vi "PDF Konfig CG.vi"(8 "error in (no error)":errorcluster caption="Fehler (Eingang, kein Fehler)", 11 "seconds since 1Jan1904":timestamp) -> (0 "error out":errorcluster caption="Fehler (Ausgang)")   [LabVIEW 2020, in "Erweiterte Konfig.lvlib" / "CG-Check Konfig.lvlib"]
uses:
  CG-Check Konfig.lvlib
  Schedule Modul/Aktion FGV Testdaten sammeln.ctl
  Sprachverwaltung/FGV Aktion Tabelle zerlegen.ctl
  Linearisierung V2/Protokoll/Protokoll.lvlib
  Schedule Modul/Schedule Modul.lvlib
  Sprachverwaltung/Sprachverwaltung.lvlib
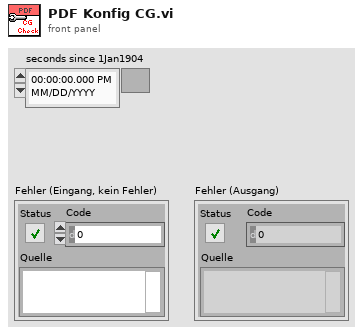
[diagram p1: front panel]
types:
  T1 = typedef "Sprachverwaltung.lvlib/FGV Aktion Tabelle zerlegen.ctl" = enum16{"laden", "vereinzeln", "speichern"}
  T2 = typedef "Schedule Modul.lvlib/Aktion FGV Testdaten sammeln.ctl" = enum16{"lesen", "Dichtheitstest", "CalGasTest", "T90", "Kalibrieren", "init", "Kalender Daten"}
  T3 = typedef "Schedule Modul.lvlib/Ergebnis CalGas Test.ctl" = cluster{"Istwerte":string[][], "Auswertung":string[][][], "Fehler":bool[], "Abweichung in %":string[][], "Spanauswahl":i32[]}
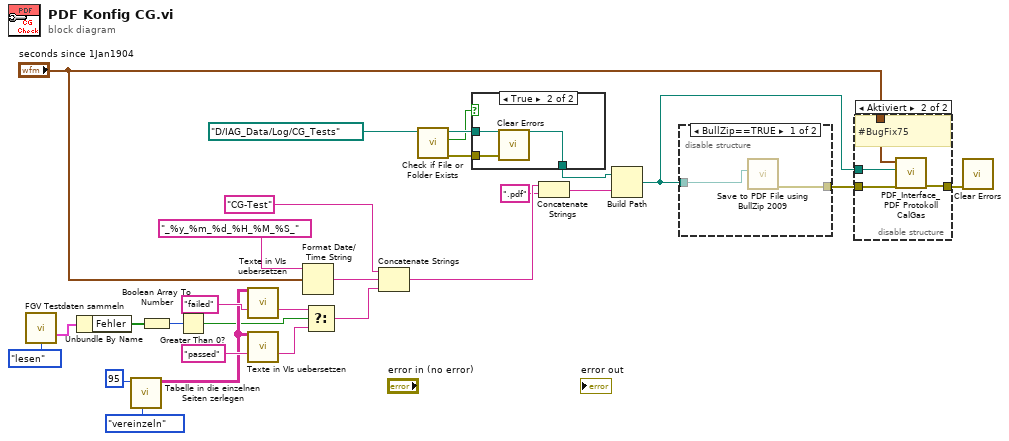
[diagram p0: block diagram]
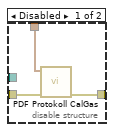
[diagram p2: hidden frame]
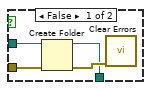
[diagram p3: hidden frame]
diagram:
  n1 = call "FGV Testdaten sammeln.vi"("Aktion"=Aktion_FGV_Testdaten_sammeln."lesen") -> ("Ergebnis CalGas Test"=w16:T3)  [unwired: 9 in, 5 out]
  n2 = Unbundle By Name(w16) -> ("Fehler"=w15:bool[])
  n3 = call "Tabelle in die einzelnen Seiten zerlegen.vi"("Aktion"=FGV_Aktion_Tabelle_zerlegen."vereinzeln", "Index (Seite)"=95) -> ("Sprachliste"=w4:string[][])  [unwired: 7 in, 2 out]
  n4 = Boolean Array To Number(Boolean array=w15) -> (number=w14:u32)
  n5 = Greater Than 0?(x=w14) -> (x > 0?=w3:bool)
  n6 = call "Texte in VIs uebersetzen.vi"("Sprachliste"=w4, "String zum Übersetzen"="failed" ("String")) -> ("String zum Übersetzen"=w6:string)  [unwired: 9 in, 4 out]
  n7 = call "Texte in VIs uebersetzen.vi"("Sprachliste"=w4, "String zum Übersetzen"="passed" ("String")) -> ("String zum Übersetzen"=w5:string)  [unwired: 9 in, 4 out]
  n8 = Format Date/Time String(time format string (%c)="_%y_%m_%d_%H_%M_%S_" ("Zeitformatierungs-String (%c)"), seconds (now)="seconds since 1Jan1904") -> (date/time string=w21:string)  [unwired: 1 in]
  n9 = Select(t=w6, s=w3, f=w5) -> (s? t:f=w2:string)
  n10 = Concatenate Strings("CG-Test" ("String"), w21, w2) -> (w23:string)
  n11 = call <vilib>:"Check if File or Folder Exists.vi"("path"=path "D:/IAG_Data/Log/CG_Tests" ("Pfad:")) -> ("error out"=w28:errorcluster, "file or folder exists?"=w25:bool, "dup path"=w26:path)  [unwired: 8 in]
  n12 = case shown="True" w25 {
    tunnel: w26 -> [w32 w34]
    tunnel: [w30 w34] -> w27
    tunnel: w28 -> [w29 w33]
    frame False {
      n13 = Create Folder(path (use dialog)=w32, error in=w29) -> (created path=w30:path, error out=w31:errorcluster)  [unwired: 1 in, 1 out]
      n14 = call <vilib>:"Clear Errors.vi"("error in (no error)"=w31) -> ()  [unwired: 5 in, 2 out]
    }
    frame True {
      n15 = call <vilib>:"Clear Errors.vi"("error in (no error)"=w33) -> ()  [unwired: 5 in, 2 out]
    }
  }
  n16 = Concatenate Strings(w23, ".pdf" ("String")) -> (w18:string)
  n17 = Build Path(base path=w27, name or relative path=w18) -> (appended path=w1:path)
  n18 = disable-structure shown="BullZip==TRUE" {
    disable-tunnel: [w36 _] -> w13
    disable-tunnel: w1 -> [w35 _]
    frame condition #0 {
      n19 = call "Save to PDF File using BullZip 2009.vi"("Save PDF File Path"=w35) -> ("error out"=w36:errorcluster)  [unwired: 10 in]
    }
    frame condition #1 (active) {
    }
  }
  n20 = disable-structure shown="Aktiviert" {
    disable-tunnel: w13 -> [w39 w42]
    disable-tunnel: [w38 w41] -> w12
    disable-tunnel: "seconds since 1Jan1904" -> [w37 w43]
    disable-tunnel: w1 -> [_ w40]
    frame Disabled {
      n21 = call "PDF Protokoll CalGas.vi"("error in (no error)"=w39, "Zeitstempel"=w37) -> ("error out"=w38:errorcluster)  [unwired: 9 in]
    }
    frame Enabled {
      # "#BugFix75"
      n22 = call "PDF_Interface_PDF Protokoll CalGas.vi"("error in (no error)"=w42, "Save PDF File Path"=w40, "Zeitstempel"=w43) -> ("error out"=w41:errorcluster)  [unwired: 8 in]
    }
  }
  n23 = call <vilib>:"Clear Errors.vi"("error in (no error)"=w12) -> ()  [unwired: 5 in, 2 out]
